vi "Expand.vi"(8 "error in (no error)":errorcluster, 9 "CurrentLinkedNodes":refnum<data-value>[](array[refnum]), 10 "NodeToExpand in":refnum<data-value>, 11 "SudukuBoard in":refnum<class "SudokuBoard.lvclass">) -> (0 "error out":errorcluster, 1 "NodesToLinkAndExpand":refnum<data-value>[](array[refnum]), 2 "NodeToExpand out":refnum<data-value>, 3 "SudukuBoard out":refnum<class "SudokuBoard.lvclass">)   [LabVIEW 2009, in "SudokuBoard.lvclass"]
uses:
  SudokuBoard.lvclass
  GraphNode/GraphNode.lvclass
  SudukuState/SudokuState.lvclass
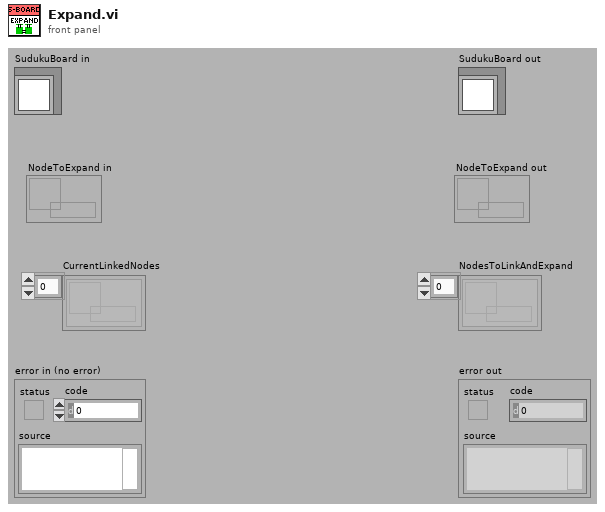
[diagram p1: front panel]
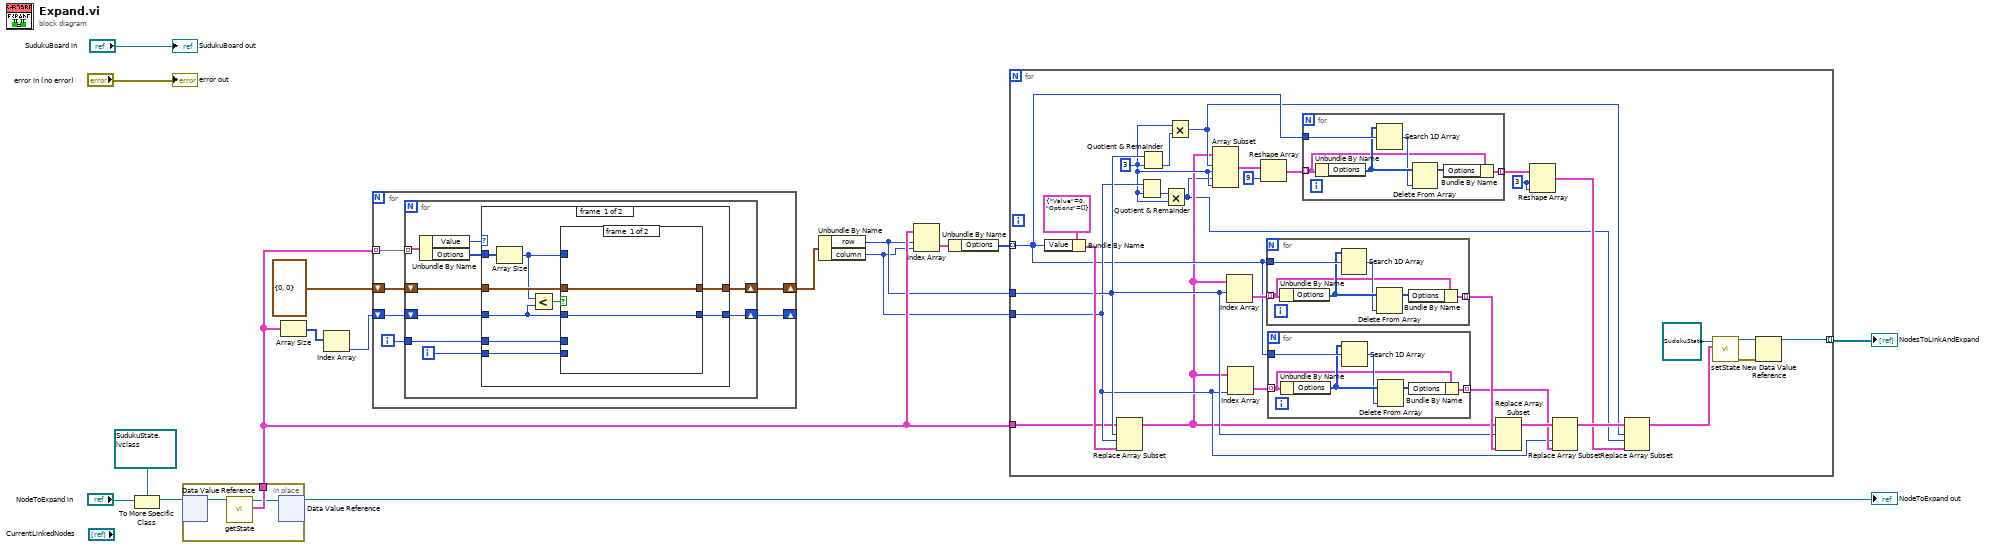
[diagram p0: block diagram]
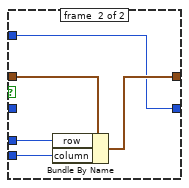
[diagram p2: hidden frame]
diagram:
  n1 = To More Specific Class(target class=refnum<data-value> refnum ("data value reference"), reference="NodeToExpand in") -> (specific class reference=w13:refnum<data-value>)  [unwired: 1 in, 1 out]
  n2 = in-place {
    in-place-border: [w18] -> w5
    n3 = in-place-dvr #1(w13) -> (w19:refnum<class "SudokuState.lvclass">)  [unwired: 1 out]
    n4 = call "getState.vi"("SudukuState in"=w19) -> ("State"=w18:cluster{"Value":i32, "Options":i32[]}[][], "SudukuState out"=w17:refnum<class "SudokuState.lvclass">)  [unwired: 8 in, 1 out]
    n5 = in-place-dvr #1(w17) -> (→"NodeToExpand out":refnum<data-value>)  [unwired: 1 out]
  }
  n6 = Array Size(array=w5) -> (size(s)=w11:i32[])
  n7 = Index Array(array=w11) -> (element=w10:i32)  [unwired: 1 in]
  n8 = for {
    tunnel: w5 -> [w23] mode=indexing
    shift-right: [w21] -> w7
    shift-left: cluster{"row":i32, "column":i32} {"row"=0, "column"=0} -> [w25]
    shift-right: [w20] -> _
    shift-left: w10 -> [w24]
    i -> [w22]
    n9 = for {
      shift-right: [w29] -> w21
      shift-left: w25 -> [w32]
      shift-right: [w28] -> w20
      shift-left: w24 -> [w31]
      tunnel: w23 -> [w34] mode=indexing
      tunnel: w22 -> [w27]
      i -> [w26]
      n10 = Unbundle By Name(w34) -> ("Value"=w33:i32, "Options"=w30:i32[])
      n11 = case shown="0" w33 {
        tunnel: w32 -> [w41 w52]
        tunnel: w31 -> [w39 w51]
        tunnel: w30 -> [w43 _]
        tunnel: [w40 w52] -> w29
        tunnel: [w38 w51] -> w28
        tunnel: w27 -> [w36 _]
        tunnel: w26 -> [w35 _]
        frame #0 {
          n12 = Array Size(array=w43) -> (size(s)=w37:i32)
          n13 = Less?(x=w37, y=w39) -> (x < y?=w42:bool)
          n14 = case shown="True" w42 {
            tunnel: w41 -> [w45 w50]
            tunnel: [w45 w49] -> w40
            tunnel: w39 -> [w44 _]
            tunnel: [w44 w48] -> w38
            tunnel: w37 -> [_ w48]
            tunnel: w36 -> [_ w47]
            tunnel: w35 -> [_ w46]
            frame #0 {
            }
            frame #1 {
              n15 = Bundle By Name(cluster=w50, "row"=w47, "column"=w46) -> (w49:cluster{"row":i32, "column":i32})
            }
          }
        }
        frame #1 {
        }
      }
    }
  }
  n16 = Unbundle By Name(w7) -> ("row"=w3:i32, "column"=w2:i32)
  n17 = Index Array(array=w5, index (row)=w3, index (col)=w2) -> (element=w4:cluster{"Value":i32, "Options":i32[]})
  n18 = Unbundle By Name(w4) -> ("Options"=w6:i32[])
  n19 = for {
    tunnel: w6 -> [w66] mode=indexing
    tunnel: w5 -> [w56]
    tunnel: w3 -> [w73]
    tunnel: w2 -> [w72]
    tunnel: [w53] -> w1 mode=indexing
    w64 = 3 ("dimension size")
    w61 = 3 ("y")
    n20 = Bundle By Name(cluster=cluster{"Value":i32, "Options":i32[]} {"Value"=0, "Options"=[]} ("element"), "Value"=w66) -> (w80:cluster{"Value":i32, "Options":i32[]})
    n21 = Replace Array Subset(array=w56, new element=w80, index (row)=w73, index (col)=w72) -> (w58:cluster{"Value":i32, "Options":i32[]}[][])
    n22 = Quotient & Remainder(x=w72, y=w61) -> (floor(x/y)=w71:i32)  [unwired: 1 out]
    n23 = Quotient & Remainder(x=w73, y=w61) -> (floor(x/y)=w70:i32)  [unwired: 1 out]
    n24 = Multiply(x=w71, y=w61) -> (x*y=w57:i32)
    n25 = Multiply(x=w61, y=w70) -> (x*y=w62:i32)
    n26 = Array Subset(array=w58, index (row)=w62, length (row)=w61, index (col)=w57, length (col)=w61) -> (w69:cluster{"Value":i32, "Options":i32[]}[][])
    n27 = Index Array(array=w58, index (row)=w73) -> (element=w79:cluster{"Value":i32, "Options":i32[]}[])  [unwired: 1 in]
    n28 = Index Array(array=w58, index (col)=w72) -> (element=w78:cluster{"Value":i32, "Options":i32[]}[])  [unwired: 1 in]
    n29 = Reshape Array(w69, 9 ("dimension size")) -> (w68:cluster{"Value":i32, "Options":i32[]}[])
    n30 = for {
      tunnel: w79 -> [w96] mode=indexing
      tunnel: w66 -> [w99]
      tunnel: [w94] -> w76 mode=indexing
      n31 = Unbundle By Name(w96) -> ("Options"=w98:i32[])
      n32 = Search 1D Array(1D array=w98, element=w99) -> (index of element=w97:i32)  [unwired: 1 in]
      n33 = Delete From Array(array=w98, index=w97) -> (array with subset deleted=w95:i32[])  [unwired: 1 in, 1 out]
      n34 = Bundle By Name(cluster=w96, "Options"=w95) -> (w94:cluster{"Value":i32, "Options":i32[]})
    }
    n35 = for {
      tunnel: w78 -> [w90] mode=indexing
      tunnel: w66 -> [w93]
      tunnel: [w88] -> w75 mode=indexing
      n36 = Unbundle By Name(w90) -> ("Options"=w92:i32[])
      n37 = Search 1D Array(1D array=w92, element=w93) -> (index of element=w91:i32)  [unwired: 1 in]
      n38 = Delete From Array(array=w92, index=w91) -> (array with subset deleted=w89:i32[])  [unwired: 1 in, 1 out]
      n39 = Bundle By Name(cluster=w90, "Options"=w89) -> (w88:cluster{"Value":i32, "Options":i32[]})
    }
    n40 = for {
      tunnel: w68 -> [w84] mode=indexing
      tunnel: w66 -> [w87]
      tunnel: [w82] -> w65 mode=indexing
      n41 = Unbundle By Name(w84) -> ("Options"=w86:i32[])
      n42 = Search 1D Array(1D array=w86, element=w87) -> (index of element=w85:i32)  [unwired: 1 in]
      n43 = Delete From Array(array=w86, index=w85) -> (array with subset deleted=w83:i32[])  [unwired: 1 in, 1 out]
      n44 = Bundle By Name(cluster=w84, "Options"=w83) -> (w82:cluster{"Value":i32, "Options":i32[]})
    }
    n45 = Replace Array Subset(array=w58, new element=w76, index (row)=w73) -> (w77:cluster{"Value":i32, "Options":i32[]}[][])  [unwired: 1 in]
    n46 = Reshape Array(w65, w64, w64) -> (w60:cluster{"Value":i32, "Options":i32[]}[][])
    n47 = Replace Array Subset(array=w77, new element=w75, index (col)=w72) -> (w63:cluster{"Value":i32, "Options":i32[]}[][])  [unwired: 1 in]
    n48 = Replace Array Subset(array=w63, new element=w60, index (row)=w62, index (col)=w57) -> (w59:cluster{"Value":i32, "Options":i32[]}[][])
    n49 = call "setState.vi"("State"=w59, "SudukuState in"=refnum<class "SudokuState.lvclass"> refnum ("SudukuState.lvclass")) -> ("error out"=w55:errorcluster, "SudukuState out"=w54:refnum<class "SudokuState.lvclass">)  [unwired: 8 in]
    n50 = New Data Value Reference(data value=w54, error in=w55) -> (data value reference=w53:refnum<data-value>)  [unwired: 1 out]
  }
  "NodesToLinkAndExpand" <- w1
  "error out" <- "error in (no error)"
  "SudukuBoard out" <- "SudukuBoard in"
